vi "Exercise 10.1_Answer_Queue.vi"() -> ()   [LabVIEW 2010]
uses:
  <vilib>/Analysis/NI_AALBase.lvlib
  <vilib>/Analysis/3filter.llb/Bessel Filter (DBL).vi
panel:
  out "# elements in queue":i32
  in  "stop 2":bool
  out "Consumer Loop Rate (Hz)":u32
  out "Processed Data":dbl[][](graph)
  in  "stop":bool
  out "Raw Data":dbl[][](graph)
  out "Producer Loop Rate (Hz)":u32
  out "Data Produced":i32
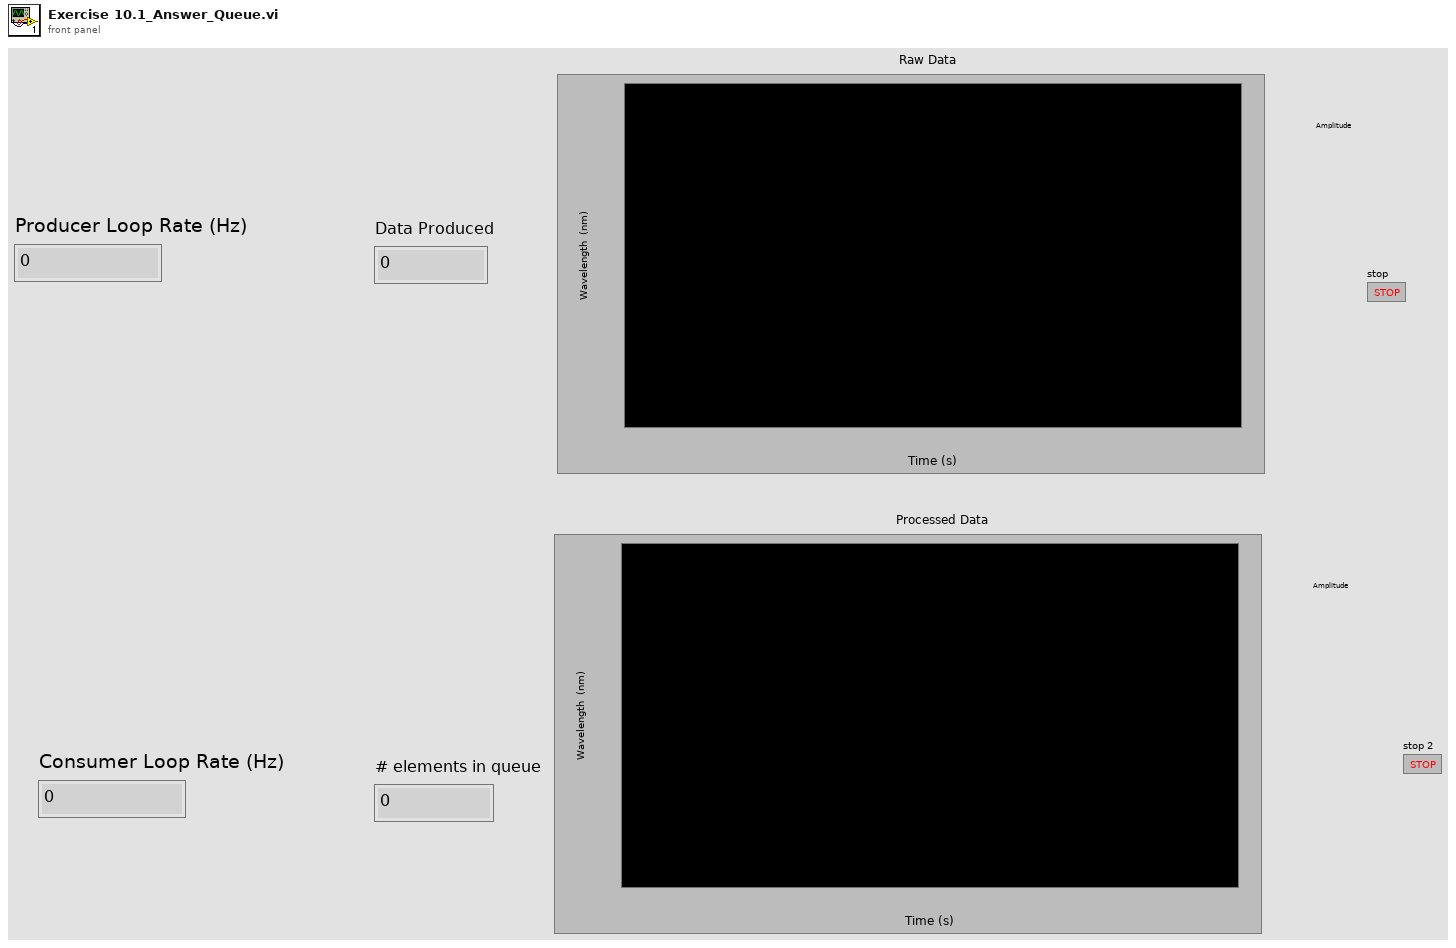
[diagram p1: front panel]
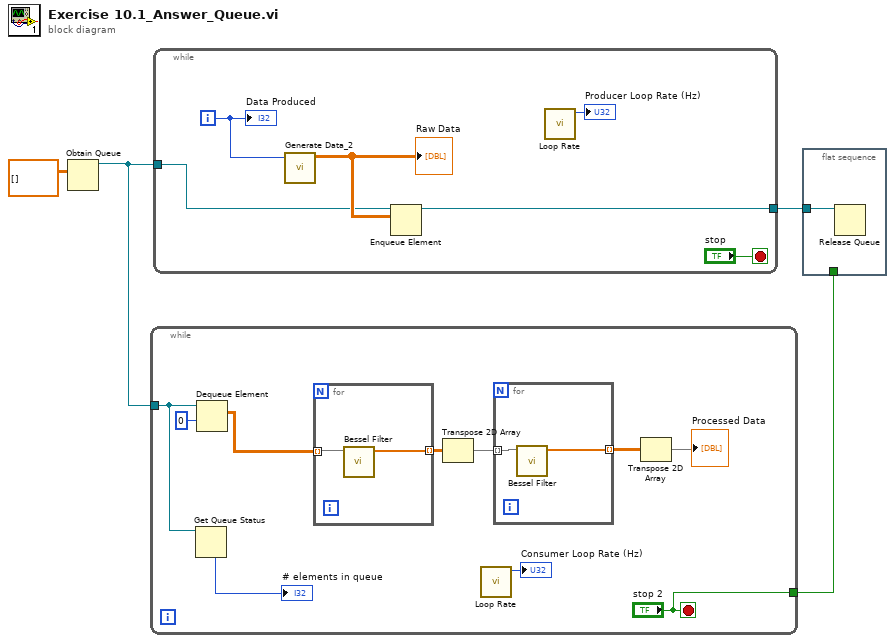
[diagram p0: block diagram]
diagram:
  n1 = Obtain Queue(element data type=dbl[][] [] ("Raw Data")) -> (queue out=w2:refnum<queue>)  [unwired: 4 in, 2 out]
  n2 = while {
    tunnel: w2 -> [w7]
    tunnel: ["stop 2"] -> w1
    stop <- "stop 2" stop-if-true
    n3 = Get Queue Status(queue=w7) -> (# elements in queue=→"# elements in queue":i32)  [unwired: 2 in, 7 out]
    n4 = Dequeue Element(queue=w7, timeout in ms (-1)=0) -> (element=w9:dbl[][])  [unwired: 1 in, 3 out]
    n5 = for {
      tunnel: w9 -> [w18] mode=indexing
      tunnel: [w17] -> w14 mode=indexing
      n6 = call-poly <vilib>:"Bessel Filter.vi"("X"=w18) -> ("Filtered X"=w17:dbl[])  [unwired: 7 in, 1 out]
    }
    n7 = Transpose 2D Array(2D array=w14) -> (transposed array=w13:dbl[][])
    n8 = call "Loop Rate.vi"() -> ("Loop Rate (Hz)"=→"Consumer Loop Rate (Hz)":u32)  [unwired: 11 in]
    n9 = for {
      tunnel: w13 -> [w16] mode=indexing
      tunnel: [w15] -> w12 mode=indexing
      n10 = call-poly <vilib>:"Bessel Filter.vi"("X"=w16) -> ("Filtered X"=w15:dbl[])  [unwired: 7 in, 1 out]
    }
    n11 = Transpose 2D Array(2D array=w12) -> (transposed array=→"Processed Data":dbl[][])
  }
  n12 = while {
    tunnel: w2 -> [w20]
    tunnel: [w19] -> w3
    i -> [w24]
    stop <- "stop" stop-if-true
    n13 = call "Generate Data_2.vi"("Input"=w24) -> ("Array out"=w21:dbl[][])  [unwired: 10 in]
    "Raw Data" <- w21
    n14 = Enqueue Element(queue=w20, element=w21) -> (queue out=w19:refnum<queue>)  [unwired: 2 in, 2 out]
    n15 = call "Loop Rate.vi"() -> ("Loop Rate (Hz)"=→"Producer Loop Rate (Hz)":u32)  [unwired: 11 in]
    "Data Produced" <- w24
  }
  n16 = flat-sequence {
    tunnel: w3 -> [w25]
    tunnel: w1 -> [_]
    frame #0 {
      n17 = Release Queue(queue=w25) -> ()  [unwired: 2 in, 3 out]
    }
  }
